vi "doTileScan.vi"(0 "Positioners (motors)":T3={"overlap"=0.5, "pos-xy_start"={"pos-x_start"=0.0, "pos-y_start"=10.0}, "pos-xy_end"={"pos-x_end"=0.06, "pos-y_end"=0.06}, "pos-xy_ref"={"pos-x_start"=0.0, "pos-y_start"=10.0}} {"pos-xy_ref"."pos-y_start" format="%.3e"; "pos-xy_ref"."pos-x_start" format="%.3e"; "pos-xy_end"."pos-y_end" format="%.3e"; "pos-xy_end"."pos-x_end" format="%.3e"; "pos-xy_start"."pos-y_start" format="%.3e"; "pos-xy_start"."pos-x_start" format="%.3e"}, 3 "IntensityGraph in":refnum<vi>, 4 "status-event":refnum<event-registration>, 5 "Image (mirrors)":T2={"image_size"=6.0, "image_xy_start"={"image-x_start"=0.0, "image-y_start"=0.0}, "pixel_dwell_ms"=100.0, "frame_size_x_px"=100, "scan_direction"=enum."0", "pos_start"=enum."bottom-left"}, 7 "Focus (Piezo)":T1={"z_start"=0.0, "z_end"=100.0, "q_steps"=100, "dwell_time_ms"=100.0}, 9 "XY Max?":bool, 14 "queue-commands":refnum<queue>, 15 "WFChart Refnum":refnum<vi>) -> ()   [LabVIEW 2014]
uses:
  <vilib>/Analysis/1siggen.llb/Ramp Pattern by Delta.vi
  <vilib>/Analysis/NI_AALBase.lvlib
panel:
  # "All distances are in mm"
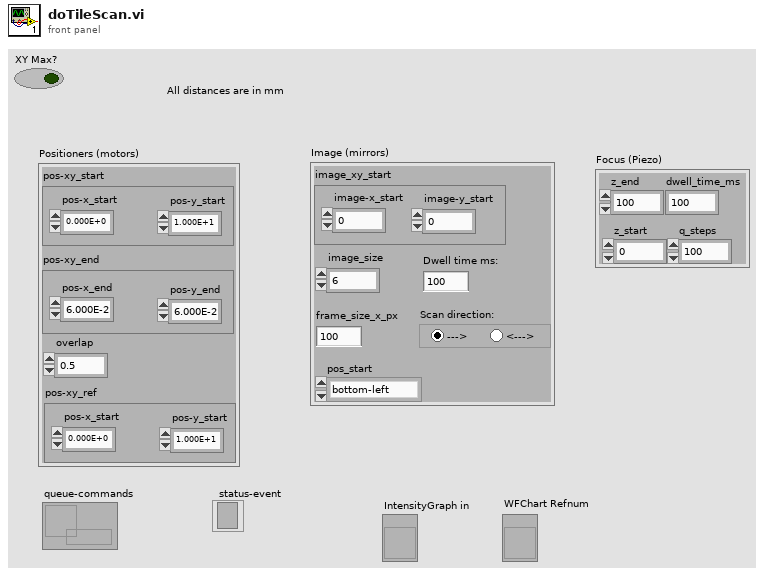
[diagram p1: front panel]
types:
  T1 = cluster{"z_start":dbl, "z_end":dbl, "q_steps":i32, "dwell_time_ms":dbl}
  T2 = cluster{"image_size":dbl, "image_xy_start":cluster{"image-x_start":dbl, "image-y_start":dbl}, "pixel_dwell_ms":dbl, "frame_size_x_px":i32, "scan_direction":enum32{"0", "1"}, "pos_start":enum32{"bottom-left", "center"}}
  T3 = cluster{"overlap":dbl, "pos-xy_start":cluster{"pos-x_start":dbl, "pos-y_start":dbl}, "pos-xy_end":cluster{"pos-x_end":dbl, "pos-y_end":dbl}, "pos-xy_ref":cluster{"pos-x_start":dbl, "pos-y_start":dbl}}
  T4 = enum16{"standby", "domove", "dostop", "exit", "status"}
  T5 = cluster{enum16{"standby", "domove", "dostop", "exit", "status"}, dbl, dbl, dbl}
  T6 = cluster{"image-x_start":dbl, "image-y_start":dbl}
  T7 = cluster{"image-x_start":dbl, "image-y_start":dbl, "z_focus":dbl, "focus_data":cluster{"z_values":dbl[], dbl[]}, "z_start":dbl, "z_end":dbl, "q_steps":i32, "dwell_time_ms":dbl}
  T8 = cluster{"x_focus":dbl, "y_focus":dbl, "z_focus":dbl, "focus_data":cluster{"z_values":dbl[], dbl[]}, "z_start":dbl, "z_end":dbl, "q_steps":i32, "dwell_time":dbl}
  T9 = cluster{"image-x_start":dbl, "image-y_start":dbl, "z-focus":dbl}
  T10 = cluster{dbl, dbl, dbl, "pos-x_start":dbl, "pos-y_start":dbl, dbl}
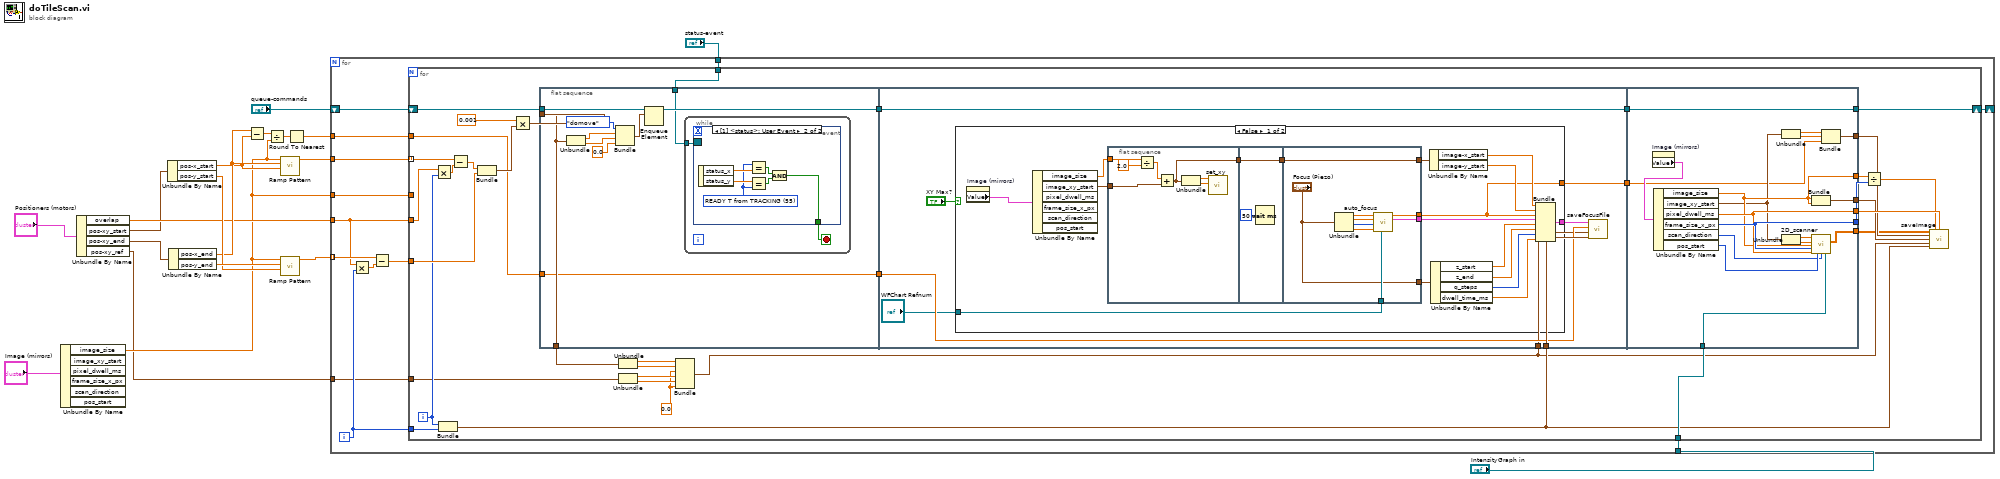
[diagram p0: block diagram]
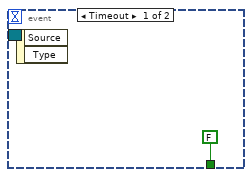
[diagram p2: hidden frame]
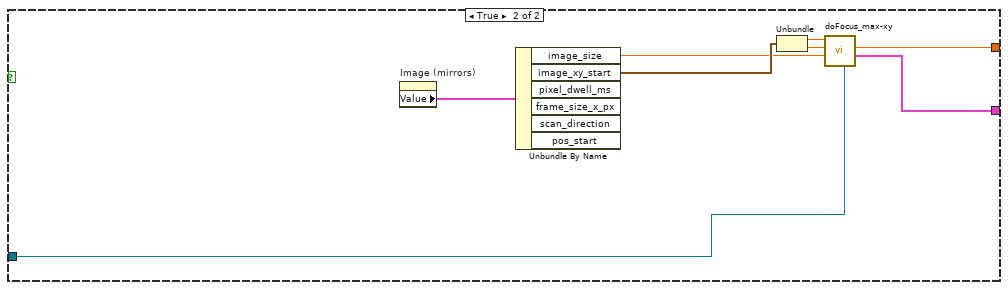
[diagram p3: hidden frame]
diagram:
  n1 = Unbundle By Name("Image (mirrors)") -> ("image_size"=w2:dbl)  [unwired: 5 out]
  n2 = Unbundle By Name("Positioners (motors)") -> ("overlap"=w6:dbl, "pos-xy_start"=w5:cluster{"pos-x_start":dbl, "pos-y_start":dbl}, "pos-xy_end"=w4:cluster{"pos-x_end":dbl, "pos-y_end":dbl}, "pos-xy_ref"=w1:cluster{"pos-x_start":dbl, "pos-y_start":dbl})
  n3 = Unbundle By Name(w5) -> ("pos-x_start"=w13:dbl, "pos-y_start"=w15:dbl)
  n4 = Unbundle By Name(w4) -> ("pos-x_end"=w14:dbl, "pos-y_end"=w16:dbl)
  n5 = Subtract(x=w14, y=w13) -> (x-y=w12:dbl)
  n6 = Divide(x=w12, y=w2) -> (x/y=w11:dbl)
  n7 = call-poly <vilib>:"Ramp Pattern.vi"("start"=w13, "end"=w14, "delta"=w2) -> ("Ramp Pattern"=w18:dbl[])  [unwired: 6 in, 2 out]
  n8 = call-poly <vilib>:"Ramp Pattern.vi"("start"=w15, "end"=w16, "delta"=w2) -> ("Ramp Pattern"=w19:dbl[])  [unwired: 6 in, 2 out]
  n9 = Round To Nearest(number=w11) -> (nearest integer value=w10:dbl)
  n10 = for {
    tunnel: w18 -> [w32]
    tunnel: w19 -> [w27] mode=indexing
    shift-right: [w30] -> _
    shift-left: "queue-commands" -> [w31]
    tunnel: w2 -> [w29]
    tunnel: "IntensityGraph in" -> [w28]
    tunnel: w6 -> [w25]
    tunnel: w10 -> [w22]
    tunnel: "status-event" -> [w21]
    tunnel: w1 -> [w20]
    i -> [w23]
    n11 = Multiply(x=w25, y=w23) -> (x*y=w26:dbl)
    n12 = Subtract(x=w27, y=w26) -> (x-y=w24:dbl)
    n13 = for {
      tunnel: w32 -> [w60] mode=indexing
      shift-right: [w66] -> w30
      shift-left: w31 -> [w67]
      tunnel: w29 -> [_]
      tunnel: w28 -> [w40]
      tunnel: w25 -> [w57]
      tunnel: w24 -> [w56]
      tunnel: w23 -> [w54]
      tunnel: w22 -> [w48]
      tunnel: w21 -> [w41]
      tunnel: w20 -> [w35]
      i -> [w55]
      w36 = 0.0
      n14 = Multiply(x=w57, y=w55) -> (x*y=w58:dbl)
      n15 = Bundle(w55, w54) -> (w39:cluster{i32, i32})  [unwired: 1 in]
      n16 = Subtract(x=w60, y=w58) -> (x-y=w59:dbl)
      n17 = Bundle(w59, w56) -> (w62:cluster{dbl, dbl})  [unwired: 1 in]
      n18 = Multiply(x=0.001 ("x+y"), y=w62) -> (x*y=w63:cluster{dbl, dbl})
      n19 = flat-sequence {
        tunnel: w67 -> [w77]
        tunnel: w63 -> [w76]
        tunnel: [w70] -> w65
        tunnel: [w76] -> w51
        tunnel: w48 -> [w69]
        tunnel: [w69] -> w47
        tunnel: w41 -> [w68]
        tunnel: w65 -> [w94]
        tunnel: [w94] -> w64
        tunnel: w39 -> [w91]
        tunnel: w47 -> [w90]
        tunnel: w34 -> [w89]
        tunnel: [w87] -> w33
        tunnel: [w154] -> w66
        tunnel: w64 -> [w154]
        tunnel: [w152] -> w42
        tunnel: [w153] -> w44
        tunnel: [w145] -> w46
        tunnel: [w144] -> w50
        tunnel: [w146] -> w49
        tunnel: [w138] -> w43
        tunnel: w40 -> [w149]
        tunnel: w33 -> [w139]
        frame #0 {
          n20 = Unbundle(w76) -> (w74:dbl, w73:dbl)
          n21 = Bundle(T4."domove", w74, w73, 0.0) -> (w72:T5)  [unwired: 1 in]
          n22 = Enqueue Element(queue=w77, element=w72) -> (queue out=w70:refnum<queue>)  [unwired: 2 in, 2 out]
          n23 = while {
            tunnel: w68 -> [w79]
            stop <- w78 stop-if-true
            n24 = event shown="[1] <status>: User Event" {
              selector: w79 -> [_ _]
              dyn-events: _ -> [_ _]
              timeout: _ -> [_ _]
              tunnel: [FALSE w82] -> w78
              event Timeout {
                n25 = event-data() -> ()  [unwired: 1 in, 2 out]
              }
              event User Event {
                w81 = u32 55 items=["READY from HOMING"=50, "READY T from READY"=54, "READY T from TRACKING"=55] ("state_to_wait")
                n26 = event-data() -> ("status_x"=w86:dbl, "status_y"=w85:dbl)  [unwired: 1 in]
                n27 = Equal?(x=w81, y=w86) -> (x = y?=w83:bool)
                n28 = Equal?(x=w85, y=w81) -> (x = y?=w84:bool)
                n29 = And(x=w83, y=w84) -> (x .and. y?=w82:bool)
              }
            }
          }
        }
        frame #1 {
          n30 = case shown="False" "XY Max?" {
            tunnel: [w110 w135] -> w92
            tunnel: "WFChart Refnum" -> [w109 w131]
            tunnel: [w95 w130] -> w87
            frame False {
              n31 = property on="Image (mirrors)" class="Clust (strict)"() -> ("Value"=w103:T2)  [unwired: 2 in, 2 out]
              n32 = Unbundle By Name(w103) -> ("image_size"=w101:dbl, "image_xy_start"=w102:T6)  [unwired: 4 out]
              n33 = flat-sequence {
                tunnel: w102 -> [w114]
                tunnel: w101 -> [w116]
                tunnel: [w112] -> w100
                tunnel: w100 -> [w119]
                tunnel: [w119] -> w99
                tunnel: [w125] -> w111
                tunnel: [w124] -> w95
                tunnel: w109 -> [w123]
                tunnel: ["Focus (Piezo)"] -> w108
                tunnel: w99 -> [w122]
                tunnel: [w122] -> w98
                frame #0 {
                  n34 = Divide(x=w116, y=2.0) -> (x/y=w113:dbl)
                  n35 = Add(x=w113, y=w114) -> (x+y=w112:T6)
                  n36 = Unbundle(w112) -> ("image-x_start"=w118:dbl, "image-y_start"=w117:dbl)
                  n37 = call "set_xy.vi"("y_value_um"=w117, "x_value_um"=w118) -> ()  [unwired: 9 in, 1 out]
                }
                frame #1 {
                  n38 = Wait (ms)(milliseconds to wait=u32 50) -> ()  [unwired: 1 out]
                }
                frame #2 {
                  n39 = Unbundle("Focus (Piezo)") -> ("z_start"=w126:dbl, "z_end"=w127:dbl, "q_steps"=w128:i32, "dwell_time_ms"=w129:dbl)
                  n40 = call "auto_focus.vi"("counts"=w123, "dwell_time_ms"=w129, "q_steps"=w128, "z_end"=w127, "z_start"=w126) -> ("focus_data"=w125:cluster{"z_values":dbl[], dbl[]}, "z_focus"=w124:dbl)  [unwired: 5 in]
                }
              }
              n41 = Unbundle By Name(w98) -> ("image-x_start"=w97:dbl, "image-y_start"=w96:dbl)
              n42 = Unbundle By Name(w108) -> ("z_start"=w107:dbl, "z_end"=w106:dbl, "q_steps"=w105:i32, "dwell_time_ms"=w104:dbl)
              n43 = Bundle("image-x_start"=w97, "image-y_start"=w96, "z_focus"=w95, "focus_data"=w111, "z_start"=w107, "z_end"=w106, "q_steps"=w105, "dwell_time_ms"=w104) -> (w110:T7)  [unwired: 1 in]
            }
            frame True {
              n44 = property on="Image (mirrors)" class="Clust (strict)"() -> ("Value"=w134:T2)  [unwired: 2 in, 2 out]
              n45 = Unbundle By Name(w134) -> ("image_size"=w132:dbl, "image_xy_start"=w133:T6)  [unwired: 4 out]
              n46 = Unbundle(w133) -> ("image-x_start"=w137:dbl, "image-y_start"=w136:dbl)
              n47 = call "doFocus_max-xy.vi"("WFChart Refnum"=w131, "image_size_x_um"=w132, "pos-start_y"=w136, "pos-start_x"=w137) -> ("focus_data"=w135:T8, "z-focus"=w130:dbl)  [unwired: 6 in]
            }
          }
          n48 = call "saveFocusFile.vi"("tile_n_xy"=w91, "micro_pos-xyz"=w89, "q_tiles_x"=w90, "focus_data"=w92) -> ()  [unwired: 2 in, 1 out]
        }
        frame #2 {
          n49 = property on="Image (mirrors)" class="Clust (strict)"() -> ("Value"=w143:T2)  [unwired: 2 in, 2 out]
          n50 = Unbundle By Name(w143) -> ("image_size"=w144:dbl, "image_xy_start"=w142:T6, "pixel_dwell_ms"=w145:dbl, "frame_size_x_px"=w146:i32, "scan_direction"=w147:enum32{"0", "1"}, "pos_start"=w148:enum32{"bottom-left", "center"})
          n51 = Unbundle(w142) -> ("image-x_start"=w141:dbl, "image-y_start"=w140:dbl)
          n52 = Unbundle(w142) -> ("image-x_start"=w151:dbl, "image-y_start"=w150:dbl)
          n53 = Bundle("image_size"=w144, "image_size"=w144) -> (w153:cluster{"image_size":dbl, "image_size":dbl})  [unwired: 1 in]
          n54 = call "2D_scanner.vi"("pos-start_x"=w151, "pos-start_y"=w150, "image_size_x_um"=w144, "frame_size_x_px"=w146, "pixel_dwell_ms"=w145, "pos_start"=w148, "scan_direction"=w147, "reference"=w149) -> ("image_out"=w152:dbl[][])  [unwired: 7 in]
          n55 = Bundle("image-x_start"=w141, "image-y_start"=w140, "z-focus"=w139) -> (w138:T9)  [unwired: 1 in]
        }
      }
      n56 = Unbundle(w51) -> (w52:dbl, w53:dbl)
      n57 = Unbundle(w35) -> ("pos-x_start"=w38:dbl, "pos-y_start"=w37:dbl)
      n58 = Bundle(w52, w53, w36, "pos-x_start"=w38, "pos-y_start"=w37, w36) -> (w34:T10)  [unwired: 1 in]
      n59 = Divide(x=w50, y=w49) -> (x/y=w45:dbl)
      n60 = call "saveImage.vi"("image"=w42, "image-step_size"=w45, "image-dwell_time"=w46, "image_start_xyz"=w43, "image_size_xy"=w44, "micro_pos-xyz"=w34, "tile_n_xy"=w39) -> ()  [unwired: 8 in, 1 out]
    }
  }
